vi "Deserialisierer Empfangsdaten.vi"(11 "CAN Daten":T1[](array[typedef]) {"payload" format="%x"; "timestamp" format="%<%.7X\n%x>T"; "type" items=["CAN Data"=0, "CAN Remote"=1, "CAN Bus Error"=2, "CAN 2.0 Data"=8, "CAN FD Data"=16, "CAN FD+BRS Data"=24, "J1939 Data"=192, "Delay"=224, "Log Trigger"=225, "Start Trigger"=226]; "identifier" format="%x"}) -> ()   [LabVIEW 2020, in "CAN Interface.lvlib"]
uses:
  CAN Interface.lvlib
  <vilib>/xnet/xnet.llb/XNET Frame CAN.ctl
  <vilib>/xnet/xnet.llb/XNET Frame Type CAN.ctl
  FGV CAN Daten Aktionen.ctl
  Allgemein/Allgemein.lvlib
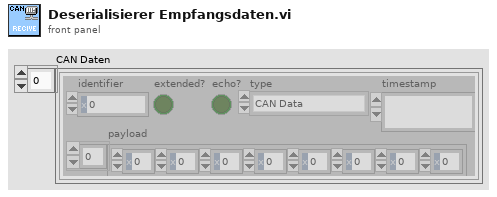
[diagram p1: front panel]
types:
  T1 = typedef "XNET Frame CAN.ctl" = cluster{"timestamp":timestamp, "payload":u8[], "identifier":u32, "type":T2, "extended?":bool, "echo?":bool}
  T2 = typedef "XNET Frame Type CAN.ctl" = u8
  T3 = typedef "CAN Interface.lvlib/FGV CAN Daten Aktionen.ctl" = enum16{"lesen", "Daten", "Konfig", "laden", "speichern", "Status"}
  T4 = typedef "CAN Konfig.lvlib/Konfig Daten PC.ctl" = cluster{"Baude Rate":T5, "COM state":u8, "Frame-ID FTIR Start":u32, "Frame-ID FTIR End":u32, "Frame-ID Status Start":u32, "Frame-ID Status End":u32, "Zustand Information":u32, "Aktion":u32, "Frame-ID FTIR Arry":u32[], "Frame-ID Status Arry":u32[], "GPS Start":u32, "Interface":refnum<k21>}
  T5 = typedef "CAN Interface.lvlib/Baude Rate.ctl" = u32
  T6 = enum16{"big-endian, network order", "native, host order", "little-endian"}
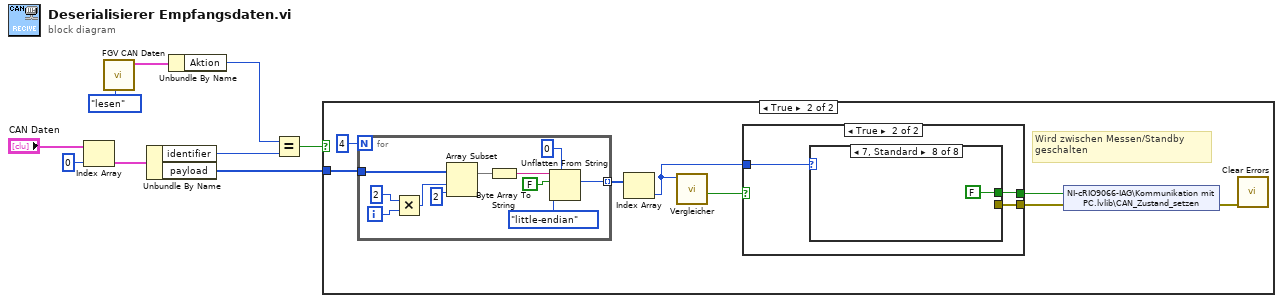
[diagram p0: block diagram]
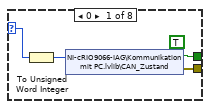
[diagram p4: hidden frame]
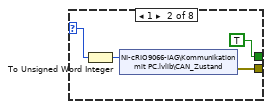
[diagram p5: hidden frame]
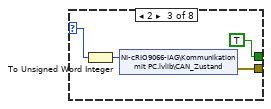
[diagram p6: hidden frame]
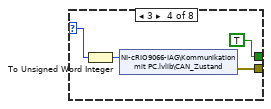
[diagram p7: hidden frame]
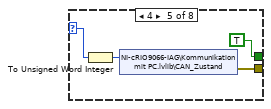
[diagram p8: hidden frame]
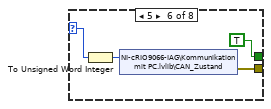
[diagram p9: hidden frame]
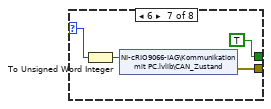
[diagram p10: hidden frame]
diagram:
  n1 = Index Array(array="CAN Daten", index=0 ("Index")) -> (element=w6:T1)
  n2 = call "FGV CAN Daten.vi"("Aktionen"=FGV_CAN_Daten_Aktionen."lesen") -> ("Konfig Daten"=w8:T4)  [unwired: 8 in, 2 out]
  n3 = Unbundle By Name(w6) -> ("identifier"=w1:u32, "payload"=w4:u8[])
  n4 = Unbundle By Name(w8) -> ("Aktion"=w2:u32)
  n5 = Equal?(x=w2, y=w1) -> (x = y?=w3:bool)
  n6 = case shown="True" w3 {
    tunnel: w4 -> [_ w16]
    frame False {
    }
    frame True {
      # "Wird zwischen Messen/Standby geschalten"
      n7 = for {
        N: 4 -> [_]
        tunnel: w16 -> [w58]
        tunnel: [w51] -> w15 mode=indexing
        i -> [w61]
        n8 = Multiply(x=2, y=w61) -> (x*y=w59:i32)
        n9 = Array Subset(array=w58, index=w59, length=2 ("Länge")) -> (w52:u8[])
        n10 = Byte Array To String(unsigned byte array=w52) -> (string=w53:string)
        n11 = Unflatten From String(type=i16 0, binary string=w53, data includes array or string size? (T)=FALSE ("Enthält Array- oder String-Größe? (T)"), byte order (0:big-endian, network order)=T6."little-endian" ("Byte-Reihenfolge (0:Big-Endian, Netzwerkreihenfolge)")) -> (value=w51:i16)  [unwired: 1 in, 2 out]
      }
      n12 = Index Array(array=w15) -> (element=w12:i16)  [unwired: 1 in]
      n13 = call "Vergleicher.vi"("Numerisch"=w12) -> ("Änderung"=w11:bool)  [unwired: 10 in]
      n14 = case shown="True" w11 {
        selector: w11 -> [w18 _]
        tunnel: [_ w21] -> w13
        tunnel: w12 -> [_ w20]
        tunnel: [w18 w19] -> w10
        frame False {
        }
        frame True {
          n15 = case shown="7, Standard" w20 {
            selector: w20 -> [w24 w28 w32 w36 w40 w44 w48 _]
            tunnel: [w25 w29 w33 w37 w41 w45 w49 _] -> w21
            tunnel: [TRUE TRUE TRUE TRUE TRUE TRUE TRUE FALSE] -> w19
            frame 0 {
              n16 = To Unsigned Word Integer(number=w24) -> (unsigned 16bit integer=w23:u16)
              n17 = shared-variable "NI-cRIO9066-IAG\\Kommunikation mit PC.lvlib\\CAN_Zustand"(w23) -> (error out=w25:errorcluster)  [unwired: 1 in]
            }
            frame 1 {
              n18 = To Unsigned Word Integer(number=w28) -> (unsigned 16bit integer=w27:u16)
              n19 = shared-variable "NI-cRIO9066-IAG\\Kommunikation mit PC.lvlib\\CAN_Zustand"(w27) -> (error out=w29:errorcluster)  [unwired: 1 in]
            }
            frame 2 {
              n20 = To Unsigned Word Integer(number=w32) -> (unsigned 16bit integer=w31:u16)
              n21 = shared-variable "NI-cRIO9066-IAG\\Kommunikation mit PC.lvlib\\CAN_Zustand"(w31) -> (error out=w33:errorcluster)  [unwired: 1 in]
            }
            frame 3 {
              n22 = To Unsigned Word Integer(number=w36) -> (unsigned 16bit integer=w35:u16)
              n23 = shared-variable "NI-cRIO9066-IAG\\Kommunikation mit PC.lvlib\\CAN_Zustand"(w35) -> (error out=w37:errorcluster)  [unwired: 1 in]
            }
            frame 4 {
              n24 = To Unsigned Word Integer(number=w40) -> (unsigned 16bit integer=w39:u16)
              n25 = shared-variable "NI-cRIO9066-IAG\\Kommunikation mit PC.lvlib\\CAN_Zustand"(w39) -> (error out=w41:errorcluster)  [unwired: 1 in]
            }
            frame 5 {
              n26 = To Unsigned Word Integer(number=w44) -> (unsigned 16bit integer=w43:u16)
              n27 = shared-variable "NI-cRIO9066-IAG\\Kommunikation mit PC.lvlib\\CAN_Zustand"(w43) -> (error out=w45:errorcluster)  [unwired: 1 in]
            }
            frame 6 {
              n28 = To Unsigned Word Integer(number=w48) -> (unsigned 16bit integer=w47:u16)
              n29 = shared-variable "NI-cRIO9066-IAG\\Kommunikation mit PC.lvlib\\CAN_Zustand"(w47) -> (error out=w49:errorcluster)  [unwired: 1 in]
            }
            frame 7, Default {
            }
          }
        }
      }
      n30 = shared-variable "NI-cRIO9066-IAG\\Kommunikation mit PC.lvlib\\CAN_Zustand_setzen"(w10, error in=w13) -> (error out=w14:errorcluster)
      n31 = call <vilib>:"Clear Errors.vi"("error in (no error)"=w14) -> ()  [unwired: 5 in, 2 out]
    }
  }
